vi "Joystick Values.vi"() -> ()   [LabVIEW 2016]
panel:
  out "GP Right Trigger":dbl
  out "GP Left Trigger":dbl
  out "GP Right X":dbl(slide) scale=0.0..1.0
  out "GP Left X":dbl(slide) scale=0.0..1.0
  out "GP Right Y":dbl(slide) scale=0.0..1.0
  out "GP Left Y":dbl(slide) scale=0.0..1.0
  out "GP Right Stick":bool
  out "GP Left Stick":bool
  out "GP Start":bool
  out "GP Back":bool
  out "GP RB":bool
  out "GP LB":bool
  out "GP B":bool
  out "GP Y":bool
  out "GP X":bool
  out "GP A":bool
  out "Right Stick Trigger":bool
  out "Left Stick Trigger":bool
  out "Right Stick Y":dbl
  out "Left Stick Y":dbl
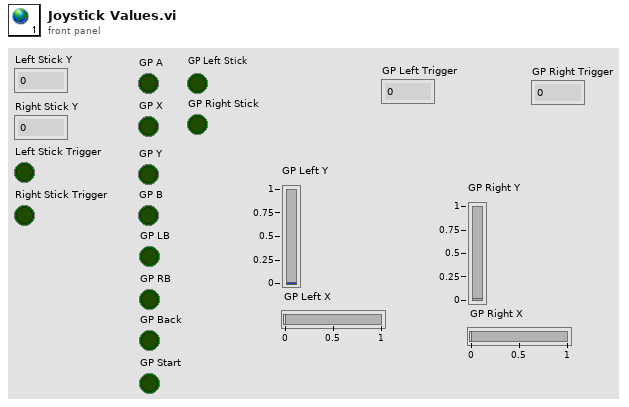
[diagram p1: front panel]
diagram:
